vi "Mouse Down.vi"(8 "error in (no error)":errorcluster, 11 "MainUI in":refnum<class "UI_Top_Customer.lvclass">) -> (0 "error out":errorcluster, 3 "MainUI out":refnum<class "UI_Top_Customer.lvclass">)   [LabVIEW 2021, in "UI_Top_Customer.lvclass"]
uses:
  UI_Top_Customer.lvclass
  UI_Top_Customer.lvclass/UI_Top_Customer.ctl
  <vilib>/ActorFramework/Actor/Actor.lvclass/Actor.ctl
  <vilib>/ActorFramework/Message Enqueuer/Message Enqueuer.lvclass/Message Enqueuer.ctl
  <vilib>/ActorFramework/Message Enqueuer/Init from Existing Queue.vi
  <vilib>/Utility/error.llb/Trim Whitespace.vi
  <vilib>/ActorFramework/Message Enqueuer/Message Enqueuer.lvclass
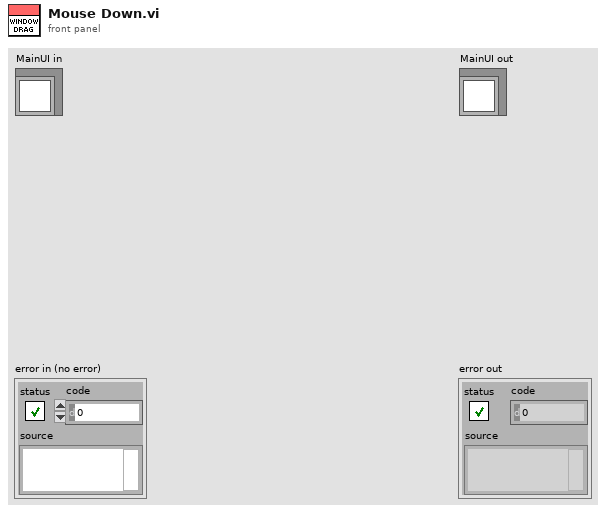
[diagram p1: front panel]
types:
  T1 = typedef "UI_Top_Customer.lvlib/UI_Top_Customer.lvclass/Pane MouseDown.ctl" = cluster{"Type":T2, "Coords":T3, "Mods":cluster{"Double Click":bool, "Menu Key":bool}, "Pane: MouseDown":bool}
  T2 = typedef "lveventtype.ctl" = enum32{"Null", "Timeout", "Annotation Menu Selection", "Annotation Menu Selection?", "App Instance Close", "App Instance Close?", "Autoscale Range Change", "Bookmark Info Change", "Cell Edit", "Cell Edit?", "Cursor Grab", "Cursor Grab?", "Cursor Menu Selection", "Cursor Menu Selection?", "Cursor Move", "Cursor Release", "Data Change", "Direction Change", "Display State Change", "Drag Ended", "Drag Enter", "Drag Leave", "Drag Over", "Drag Source Update", "Drag Starting", "Drag Starting?", "Drop", "Exec State Change", "Key Down", "Key Down?", "Key Repeat", "Key Repeat?", "Key Up", "Listbox Double Click", "Menu Activation?", "Menu Selection (App)", "Menu Selection? (App)", "Menu Selection (User)", "Mouse Down", "Mouse Down?", "Mouse Enter", "Mouse Leave", "Mouse Move", "Mouse Up", "Mouse Wheel", "NI Security User Change (App)", "Pane Size", "Panel Close", "Panel Close?", "Panel Resize", "Plot Attribute Change", "Scale Range Change", "Shortcut Menu Activation?", "Shortcut Menu Selection (App)", "Shortcut Menu Selection? (App)", "Shortcut Menu Selection (User)", "Tree Double Click", "Tree Drag", "Tree Drag?", "Tree Drop", "Tree Drop?", "Tree Item Close", "Tree Item Close?", "Tree Item Open", "Tree Item Open?", "User Event", "Value Change"}
  T3 = typedef "LVPoint32TypeDef.ctl" = cluster{"Horizontal":i32, "Vertical":i32}
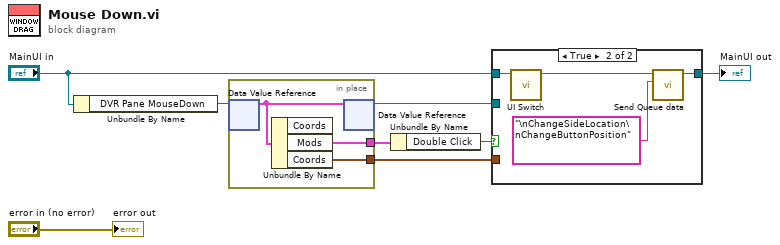
[diagram p0: block diagram]
diagram:
  n1 = Unbundle By Name("MainUI in") -> ("DVR Pane MouseDown"=w6:refnum<data-value>)
  n2 = in-place {
    in-place-border: [w10] -> w5
    in-place-border: [w9] -> w4
    n3 = in-place-dvr #1(w6) -> (w11:T1)  [unwired: 1 out]
    n4 = Unbundle By Name(w11) -> ("Mods"=w10:cluster{"Double Click":bool, "Menu Key":bool}, "Coords"=w9:T3)  [unwired: 1 out]
    n5 = in-place-dvr #1(w11) -> (w2:refnum<data-value>)  [unwired: 1 out]
  }
  n6 = Unbundle By Name(w5) -> ("Double Click"=w7:bool)
  n7 = case shown="True" w7 {
    tunnel: [w12 w16] -> w8
    tunnel: w4 -> [_ _]
    tunnel: w2 -> [_ _]
    tunnel: "MainUI in" -> [w12 w15]
    frame False {
    }
    frame True {
      n8 = call "UI Switch.vi"("UI_Top_Customer in"=w15) -> ("UI_Top_Customer out"=w13:refnum<class "UI_Top_Customer.lvclass">)  [unwired: 9 in, 1 out]
      n9 = call "Send Queue data.vi"("Elements at Back"="\nChangeSideLocation\nChangeButtonPosition", "UI_Top_Customer in"=w13) -> ("UI_Top_Customer out"=w16:refnum<class "UI_Top_Customer.lvclass">)  [unwired: 8 in, 1 out]
    }
  }
  "MainUI out" <- w8
  "error out" <- "error in (no error)"
